vi "zmq_ctx_destroy.vi"(3 "error in":errorcluster, 4 "reap? (F)":bool, 5 "context in":refnum<class "zmq_context.lvclass">) -> (0 "error out":errorcluster)   [LabVIEW 2020, in "zeromq.lvlib" / "zmq_context.lvclass"]
doc: "Terminates the <b>context</b> fed in. This is a <b>blocking</b> call, and only returns once every socket associated with the context has been terminated.\n\nBecause operations may be pending on sockets, they are given some time (ZMQ_LINGER) to finish before being shut-down by the term call.\n\nThis behaviour can be overwritten by setting <b>reap?</b> to True, which will eliminate all sockets opened by LabVIEW in this context immediately without worrying about close/blocking operations. This may result in unexpected data loss and should only be used in abort situations.\n\nDetailed API documentation: http://api.zeromq.org/3-2:zmq-ctx-destroy"
uses:
  zmq_context.lvclass
  zmq_context.lvclass/zmq_context.ctl
  Error Cluster From Error Code.vi
  zeromq.lvlib
panel:
  # "ØMQ"
  # "labview"
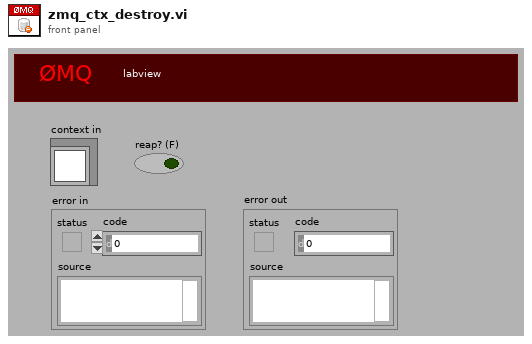
[diagram p1: front panel]
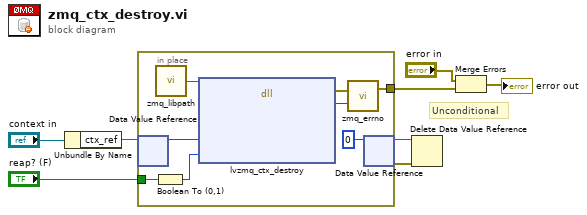
[diagram p0: block diagram]
diagram:
  # "Unconditional"
  n1 = Unbundle By Name("context in") -> ("ctx_ref"=w6:refnum<data-value>)
  n2 = in-place {
    in-place-border: [w14] -> w8
    in-place-border: "reap? (F)" -> [w12]
    n3 = in-place-dvr #1(w6) -> (w13:u64)  [unwired: 1 out]
    n4 = Boolean To (0,1)(Boolean=w12) -> (0, 1=w11:i16)
    n5 = call "zmq_libpath.vi"() -> ("path"=w9:path)
    n6 = dll-call lib="?" fn="lvzmq_ctx_destroy" ("zmq_labview.dll:lvzmq_term")(path in=w9, "ctx_obj"=w13, "flags"=w11) -> (error out=w15:errorcluster, "return"=w16:i32)  [unwired: 6 in, 1 out]
    n7 = call "zmq_errno.vi"("retval"=w16, "error in"=w15) -> ("error out"=w14:errorcluster)  [unwired: 1 out]
    n8 = in-place-dvr #1(u64 0 ("data value")) -> (w3:refnum<data-value>, w4:errorcluster)
  }
  n9 = Delete Data Value Reference(data value reference=w3, error in=w4) -> ()  [unwired: 2 out]
  n10 = Merge Errors("error in", w8) -> (→"error out":errorcluster)
